vi "Set Protocol.vi"(8 "Error In":errorcluster, 10 "Protocol in":refnum<class "Protocol Parent.lvclass">, 11 "Instrument Addon Refnum In":T1 format="%.0x") -> (0 "Error Out":errorcluster, 3 "Instrument Addon Refnum Out":T1=18446744073709551615 format="%.0x")   [LabVIEW 2018, in "Instrument Addon Scripting API.lvlib"]
doc: "Sets the Protocol for the provided Instrument Addon Custom Device. \n\nThe input Protocol object must be a child of the \"Protocol\" parent class and can be an instance of the following classes: TCP.lvclass, UDP.lvclass, VISA.lvclass, RS-xxx.lvclass, AK TCP.lvclass, AK RS-xxx.lvclass, RS-xxx to GPIB ConvBox.lvclass"
uses:
  Instrument Addon Scripting API.lvlib
  <vilib>/NI Veristand/Custom Device API/Custom Device Item Ref.ctl
  Addon/Support Libraries/Protocols.lvlibp/Protocol Parent/Protocol Parent.lvclass
  Addon/Support Libraries/Protocols.lvlibp/RS-xxx/RS-xxx.lvclass
  Addon/Addon Shared/Types/RSXXX Port Settings.ctl
  Addon/Addon Shared/Types/FG Control.ctl
  Addon/Support Libraries/Protocols.lvlibp/AK RS-xxx/AK RS-xxx.lvclass
  Addon/Support Libraries/Protocols.lvlibp/UDP/UDP.lvclass
  Addon/Addon Shared/Types/UDP Settings.ctl
  Addon/Support Libraries/Protocols.lvlibp/TCP/TCP.lvclass
  Addon/Addon Shared/Types/TCPIP Settings.ctl
  Addon/Support Libraries/Protocols.lvlibp/AK TCP/AK TCP.lvclass
  Addon/Support Libraries/Protocols.lvlibp/VISA/VISA.lvclass
  Addon/Addon Shared/Types/VISA Settings.ctl
  Addon/Support Libraries/Protocols.lvlibp/RS-xxx to GPIB ConvBox/RS-xxx to GPIB ConvBox.lvclass
  Addon/Addon Shared/Types/GPIB ConvBox Settings.ctl
  Addon/Support Libraries/Protocols.lvlibp/RS-xxx/Data Access/Read PortSettings.vi
  Addon/Addon Shared/SubVIs/Constants.vi
  <vilib>/NI Veristand/Custom Device API/NI VeriStand - Get Item Property.vi
  <vilib>/NI Veristand/Custom Device API/Get Item Property (String).vi
  <vilib>/NI Veristand/Custom Device API/Get Item Property (U32).vi
  <vilib>/NI Veristand/Custom Device API/Get Item Property (Boolean).vi
  <vilib>/NI Veristand/Custom Device API/NI VeriStand - Set Item Property.vi
  <vilib>/NI Veristand/Custom Device API/Set Item Property (String).vi
  <vilib>/NI Veristand/Custom Device API/Set Item Property (U32).vi
  <vilib>/NI Veristand/Custom Device API/Set Item Property (Boolean).vi
  <vilib>/NI/NI VeriStand Advanced SysDef API/SysDef API/SysDef.Property.Get.vi
  <vilib>/NI/NI VeriStand Advanced SysDef API/_SubVIs/SysDef.Property.Get.String.vi
  <vilib>/NI/NI VeriStand Advanced SysDef API/SysDef API/SysDef.Property.Set.vi
  <vilib>/NI/NI VeriStand Advanced SysDef API/_SubVIs/SysDef.Property.Set.String.vi
  Addon/Support Libraries/Protocols.lvlibp/UDP/Data Access/Read Local IP Address.vi
  Addon/Support Libraries/Protocols.lvlibp/UDP/Data Access/Read Local Port.vi
  Addon/Support Libraries/Protocols.lvlibp/UDP/Data Access/Read Target IP Address.vi
  Addon/Support Libraries/Protocols.lvlibp/UDP/Data Access/Read Target Port.vi
  Addon/Support Libraries/Protocols.lvlibp/TCP/Data Access/Read IP Address.vi
  Addon/Support Libraries/Protocols.lvlibp/TCP/Data Access/Read Port.vi
  Addon/Support Libraries/Protocols.lvlibp/VISA/Data Access/Read Append Write Termination Character.vi
  Addon/Support Libraries/Protocols.lvlibp/VISA/Data Access/Read Enable Termination Character.vi
  Addon/Support Libraries/Protocols.lvlibp/VISA/Data Access/Read Termination Character.vi
  Addon/Support Libraries/Protocols.lvlibp/VISA/Data Access/Read Timeout.vi
  Addon/Support Libraries/Protocols.lvlibp/VISA/Data Access/Read VISA Resource.vi
  Addon/Support Libraries/Protocols.lvlibp/RS-xxx to GPIB ConvBox/Data Access/Read Assert Ren with IFC.vi
  Addon/Support Libraries/Protocols.lvlibp/RS-xxx to GPIB ConvBox/Data Access/Read ConvBox Address.vi
  Addon/Support Libraries/Protocols.lvlibp/RS-xxx to GPIB ConvBox/Data Access/Read GPIB Address.vi
  Addon/Support Libraries/Protocols.lvlibp/RS-xxx to GPIB ConvBox/Data Access/Read IST bit sense.vi
  Addon/Support Libraries/Protocols.lvlibp/RS-xxx to GPIB ConvBox/Data Access/Read Port.vi
  Addon/Support Libraries/Protocols.lvlibp/RS-xxx to GPIB ConvBox/Data Access/Read System controller.vi
  Addon/Addon Shared/Instrument Addon Shared.lvlib
  <vilib>/NI Veristand/Custom Device API/Custom Device API.lvlib
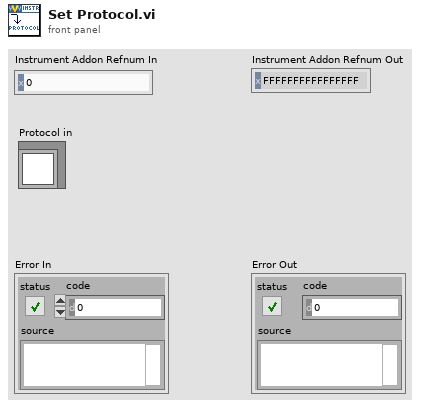
[diagram p1: front panel]
types:
  T1 = typedef "Custom Device API.lvlib/Custom Device Item Ref.ctl" = u64
  T2 = typedef "Instrument Addon Shared.lvlib/FG Control.ctl" = enum16{"Get", "Set"}
  T3 = typedef "Instrument Addon Shared.lvlib/RSXXX Port Settings.ctl" = cluster{"Port":string, "Baud Rate":u32, "Data Bits":u16, "Parity":enum16{"None", "Odd", "Even", "Mark", "Space"}, "Stop Bits":u16, "Flow Control":u16, "XON":enum16{"NUL", "SOH", "STX", "ETX", "EOT", "ENQ", "ACK", "BEL", "BS", "HT", "LF", "VT", "FF", "CR", "SO", "SI", "DLE", "DC1", "DC2", "DC3", "DC4", "NAK", "SYN", "ETB", "CAN", "EM", "SUB", "ESC", "FS", "GS", "RS", "US", "SP", "!", "\"", "#", "$", "%", "&", "'", "(", ")", "*", "+", ",", "- (-)", ".", "/", "0", "1", "2", "3", "4", "5", "6", "7", "8", "9", ":", ";", "<", "=", ">", "?", "@", "A", "B", "C", "D", "E", "F", "G", "H", "I", "J", "K", "L", "M", "N", "O", "P", "Q", "R", "S", "T", "U", "V", "W", "X", "Y", "Z", "[", "\\", "]", "^", "_", "`", "a", "b", "c", "d", "e", "f", "g", "h", "i", "j", "k", "l", "m", "n", "o", "p", "q", "r", "s", "t", "u", "v", "w", "x", "y", "z", "{", "|", "}", "~"}, "XOFF":enum16{"NUL", "SOH", "STX", "ETX", "EOT", "ENQ", "ACK", "BEL", "BS", "HT", "LF", "VT", "FF", "CR", "SO", "SI", "DLE", "DC1", "DC2", "DC3", "DC4", "NAK", "SYN", "ETB", "CAN", "EM", "SUB", "ESC", "FS", "GS", "RS", "US", "SP", "!", "\"", "#", "$", "%", "&", "'", "(", ")", "*", "+", ",", "- (-)", ".", "/", "0", "1", "2", "3", "4", "5", "6", "7", "8", "9", ":", ";", "<", "=", ">", "?", "@", "A", "B", "C", "D", "E", "F", "G", "H", "I", "J", "K", "L", "M", "N", "O", "P", "Q", "R", "S", "T", "U", "V", "W", "X", "Y", "Z", "[", "\\", "]", "^", "_", "`", "a", "b", "c", "d", "e", "f", "g", "h", "i", "j", "k", "l", "m", "n", "o", "p", "q", "r", "s", "t", "u", "v", "w", "x", "y", "z", "{", "|", "}", "~"}, "End Read on Termination Character":bool, "End Write on Termination Character":bool, "Termination Character":u8}
  T4 = typedef "Instrument Addon Shared.lvlib/UDP Settings.ctl" = cluster{"Local IP Address":string, "Local Port":u16, "Target IP Address":string, "Target Port":u16}
  T5 = typedef "Instrument Addon Shared.lvlib/TCPIP Settings.ctl" = cluster{"IP Address":string, "Port":u16}
  T6 = typedef "Instrument Addon Shared.lvlib/VISA Settings.ctl" = cluster{"VISA Resource":string, "Enable Termination Character":bool, "Termination Character":u8, "Timeout":u32, "Append Write Termination Character":bool}
  T7 = typedef "Instrument Addon Shared.lvlib/GPIB ConvBox Settings.ctl" = cluster{"Port":string, "ConvBox Address":string, "Assert Ren with IFC":bool, "System controller":bool, "IST bit sense":bool, "GPIB Address":string}
  T8 = typedef "Protocols.lvlibp/Protocol Parent.lvclass/Base Protocol Type.ctl" = enum16{"RS-XXX", "VISA", "TCPIP", "UDP", "GPIB ConvBox"}
  T9 = cluster{"Port":string, "Baud Rate":u32, "Data Bits":u16, "Parity":enum16{"None", "Odd", "Even", "Mark", "Space"}, "Stop Bits":u16, "Flow Control":u16, "XON":enum16{"NUL", "SOH", "STX", "ETX", "EOT", "ENQ", "ACK", "BEL", "BS", "HT", "LF", "VT", "FF", "CR", "SO", "SI", "DLE", "DC1", "DC2", "DC3", "DC4", "NAK", "SYN", "ETB", "CAN", "EM", "SUB", "ESC", "FS", "GS", "RS", "US", "SP", "!", "\"", "#", "$", "%", "&", "'", "(", ")", "*", "+", ",", "- (-)", ".", "/", "0", "1", "2", "3", "4", "5", "6", "7", "8", "9", ":", ";", "<", "=", ">", "?", "@", "A", "B", "C", "D", "E", "F", "G", "H", "I", "J", "K", "L", "M", "N", "O", "P", "Q", "R", "S", "T", "U", "V", "W", "X", "Y", "Z", "[", "\\", "]", "^", "_", "`", "a", "b", "c", "d", "e", "f", "g", "h", "i", "j", "k", "l", "m", "n", "o", "p", "q", "r", "s", "t", "u", "v", "w", "x", "y", "z", "{", "|", "}", "~"}, "XOFF":enum16{"NUL", "SOH", "STX", "ETX", "EOT", "ENQ", "ACK", "BEL", "BS", "HT", "LF", "VT", "FF", "CR", "SO", "SI", "DLE", "DC1", "DC2", "DC3", "DC4", "NAK", "SYN", "ETB", "CAN", "EM", "SUB", "ESC", "FS", "GS", "RS", "US", "SP", "!", "\"", "#", "$", "%", "&", "'", "(", ")", "*", "+", ",", "- (-)", ".", "/", "0", "1", "2", "3", "4", "5", "6", "7", "8", "9", ":", ";", "<", "=", ">", "?", "@", "A", "B", "C", "D", "E", "F", "G", "H", "I", "J", "K", "L", "M", "N", "O", "P", "Q", "R", "S", "T", "U", "V", "W", "X", "Y", "Z", "[", "\\", "]", "^", "_", "`", "a", "b", "c", "d", "e", "f", "g", "h", "i", "j", "k", "l", "m", "n", "o", "p", "q", "r", "s", "t", "u", "v", "w", "x", "y", "z", "{", "|", "}", "~"}, "End Read on Termination Character":bool, "End Write on Termination Character":bool, "Termination Character":u8}
  T10 = enum16{"NUL", "SOH", "STX", "ETX", "EOT", "ENQ", "ACK", "BEL", "BS", "HT", "LF", "VT", "FF", "CR", "SO", "SI", "DLE", "DC1", "DC2", "DC3", "DC4", "NAK", "SYN", "ETB", "CAN", "EM", "SUB", "ESC", "FS", "GS", "RS", "US", "SP", "!", "\"", "#", "$", "%", "&", "'", "(", ")", "*", "+", ",", "- (-)", ".", "/", "0", "1", "2", "3", "4", "5", "6", "7", "8", "9", ":", ";", "<", "=", ">", "?", "@", "A", "B", "C", "D", "E", "F", "G", "H", "I", "J", "K", "L", "M", "N", "O", "P", "Q", "R", "S", "T", "U", "V", "W", "X", "Y", "Z", "[", "\\", "]", "^", "_", "`", "a", "b", "c", "d", "e", "f", "g", "h", "i", "j", "k", "l", "m", "n", "o", "p", "q", "r", "s", "t", "u", "v", "w", "x", "y", "z", "{", "|", "}", "~"}
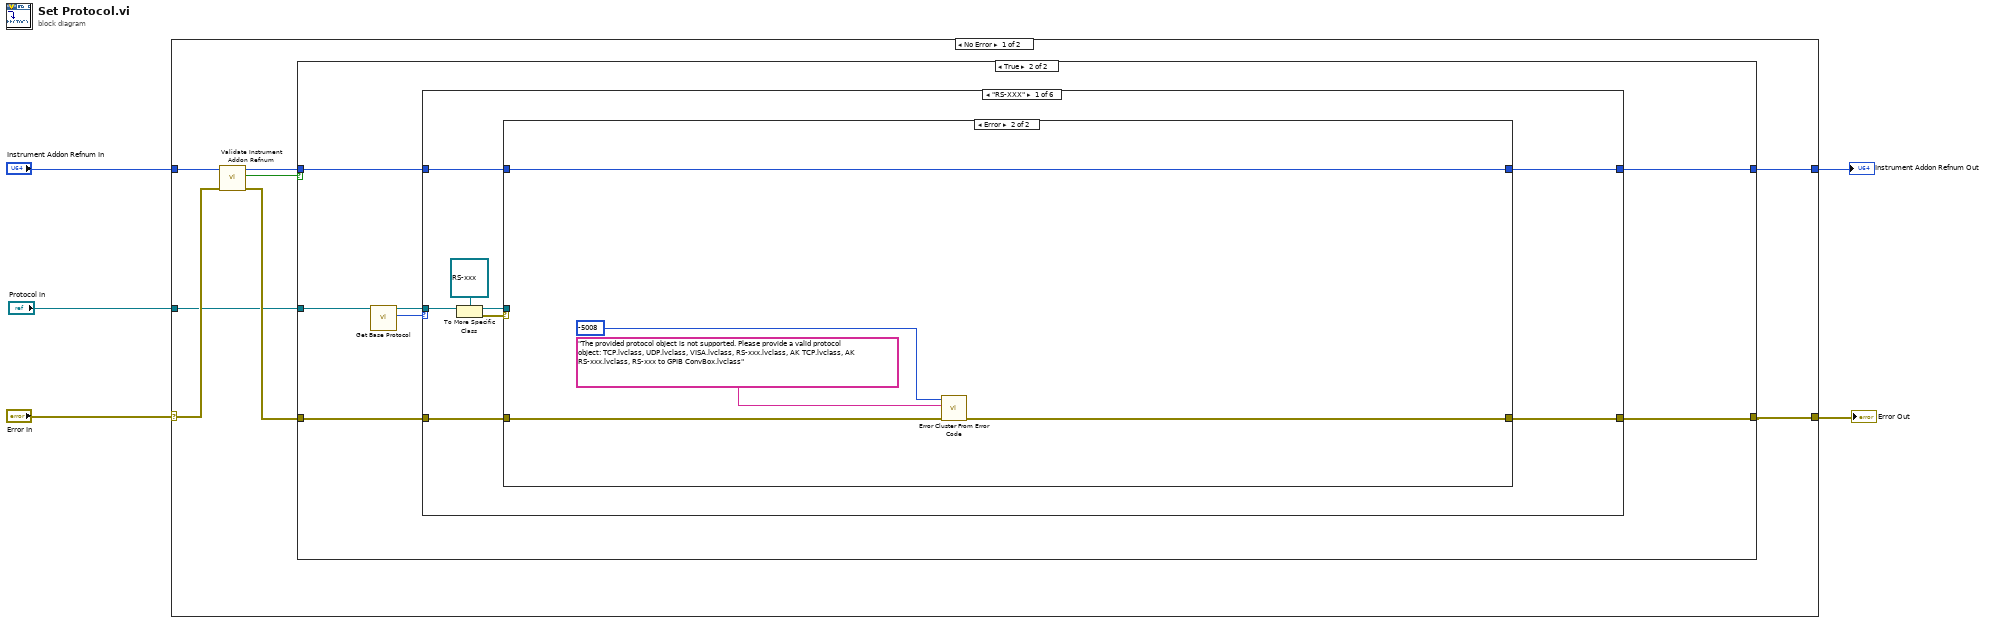
[diagram p0: block diagram]
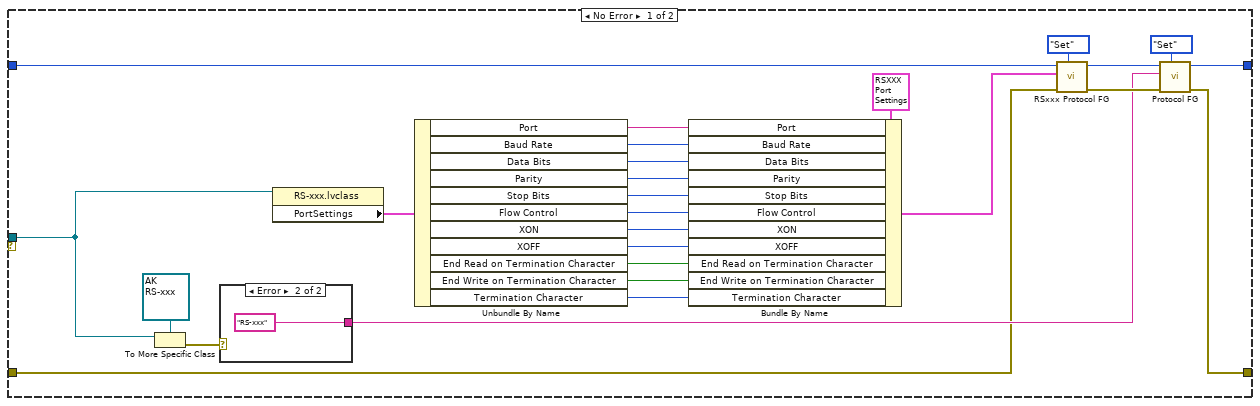
[diagram p3: hidden frame]
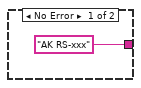
[diagram p4: hidden frame]
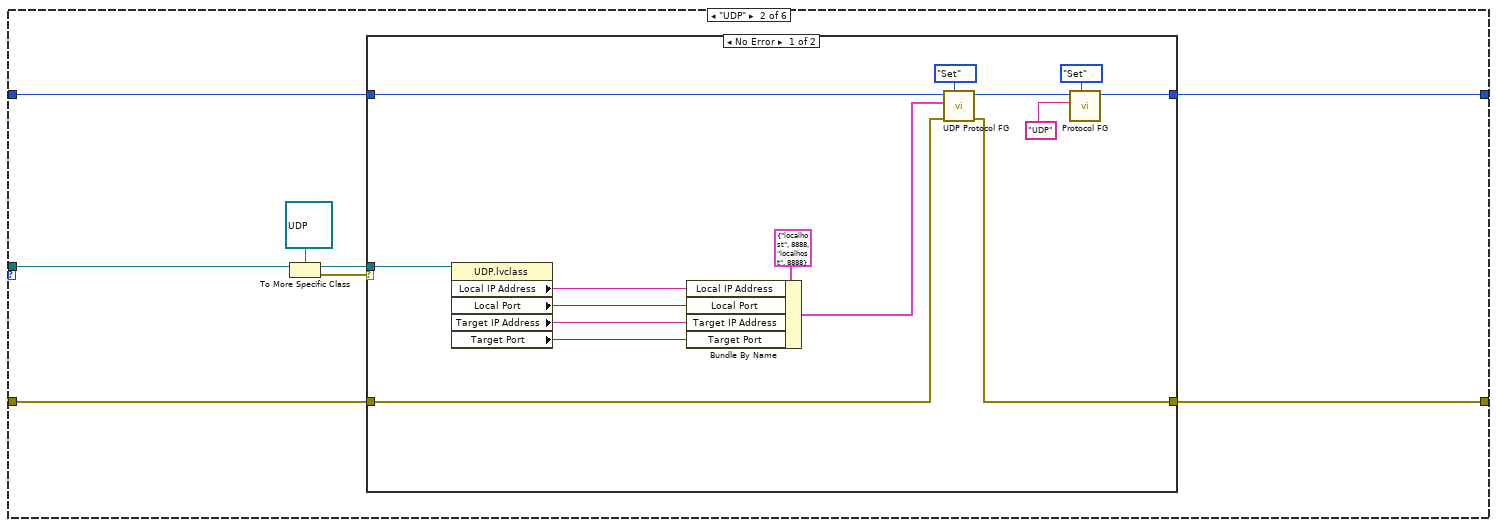
[diagram p5: hidden frame]
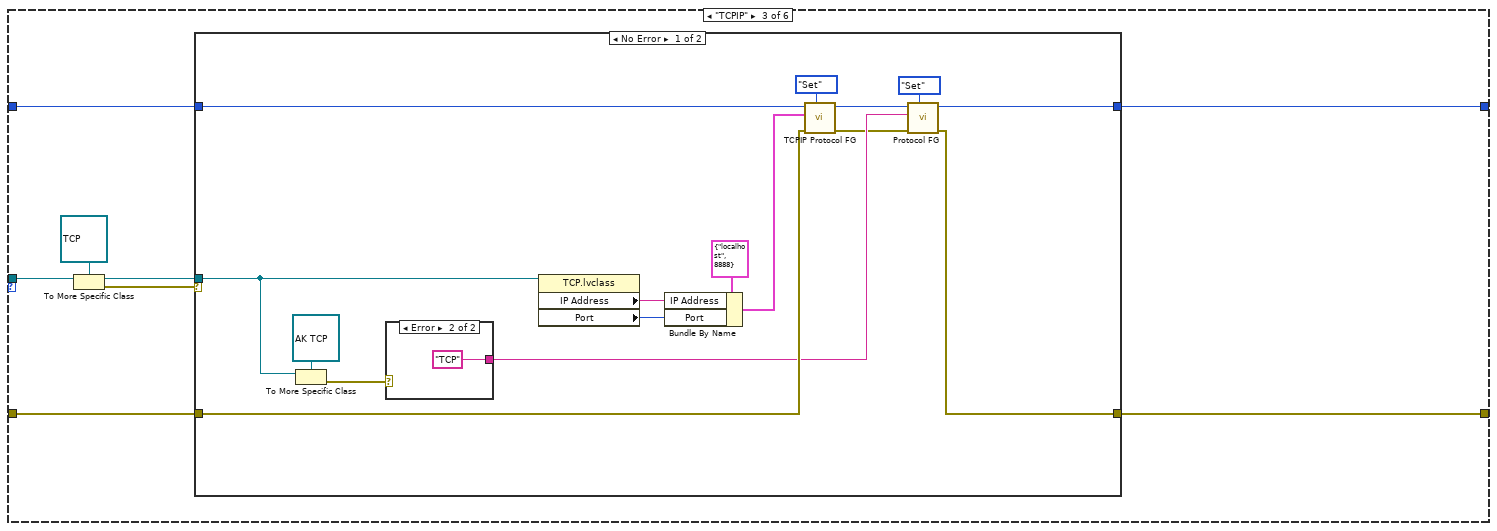
[diagram p7: hidden frame]
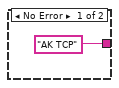
[diagram p8: hidden frame]
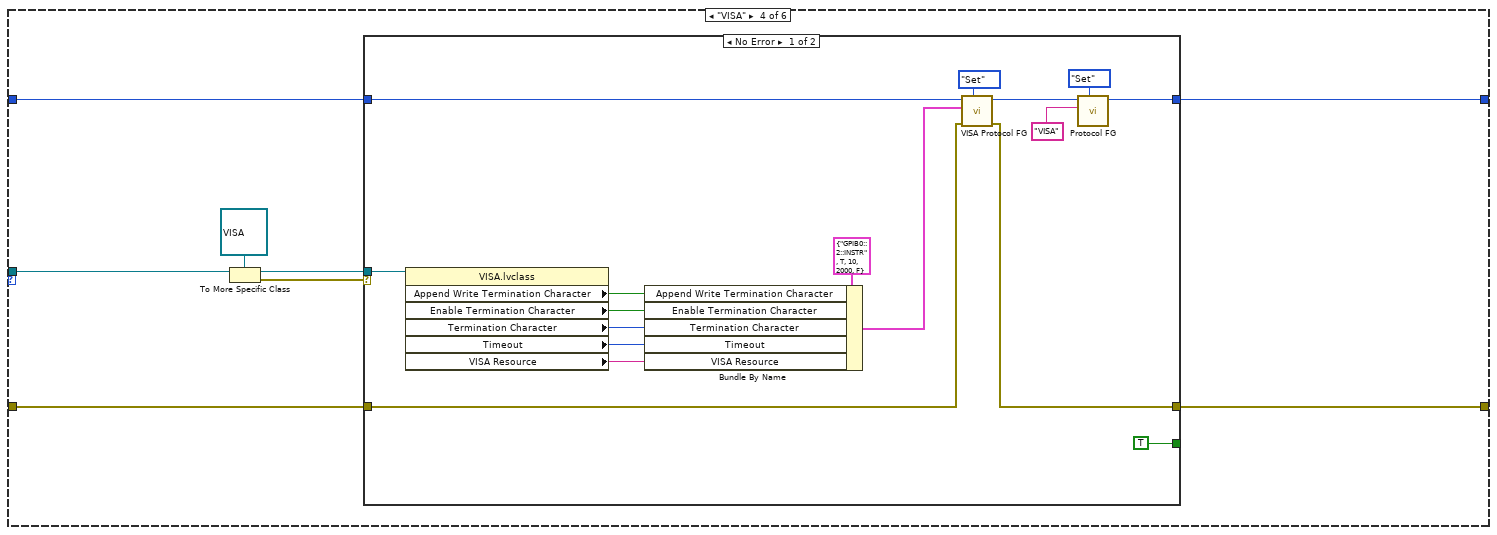
[diagram p10: hidden frame]
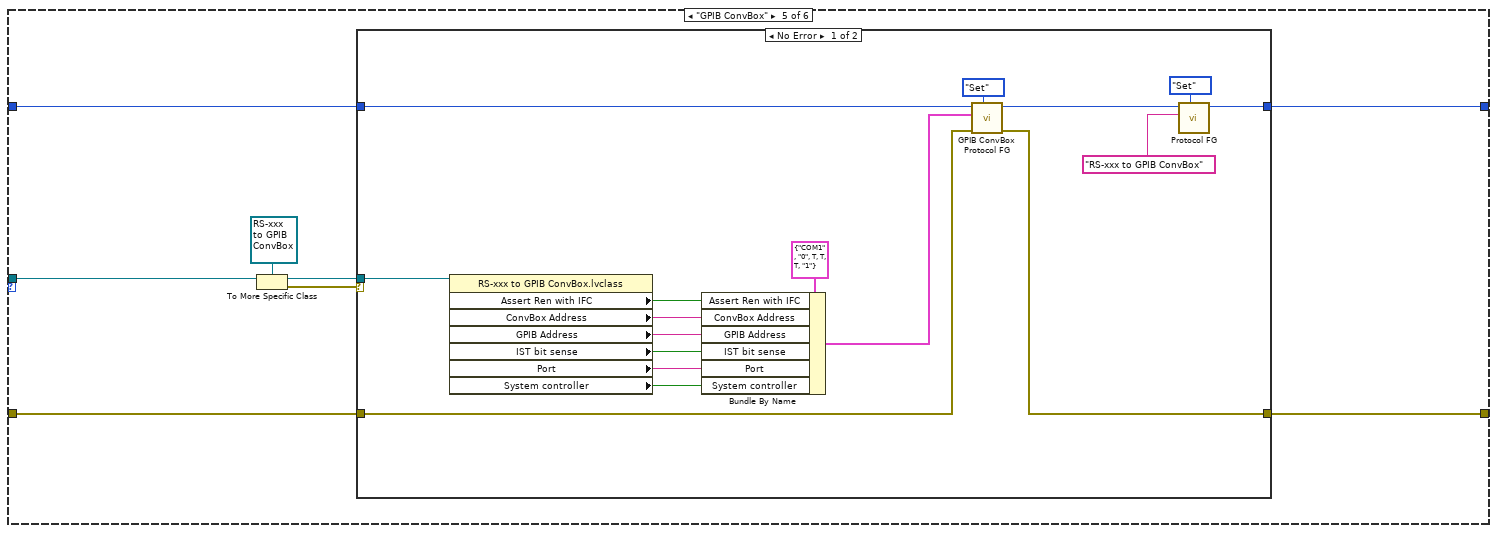
[diagram p12: hidden frame]
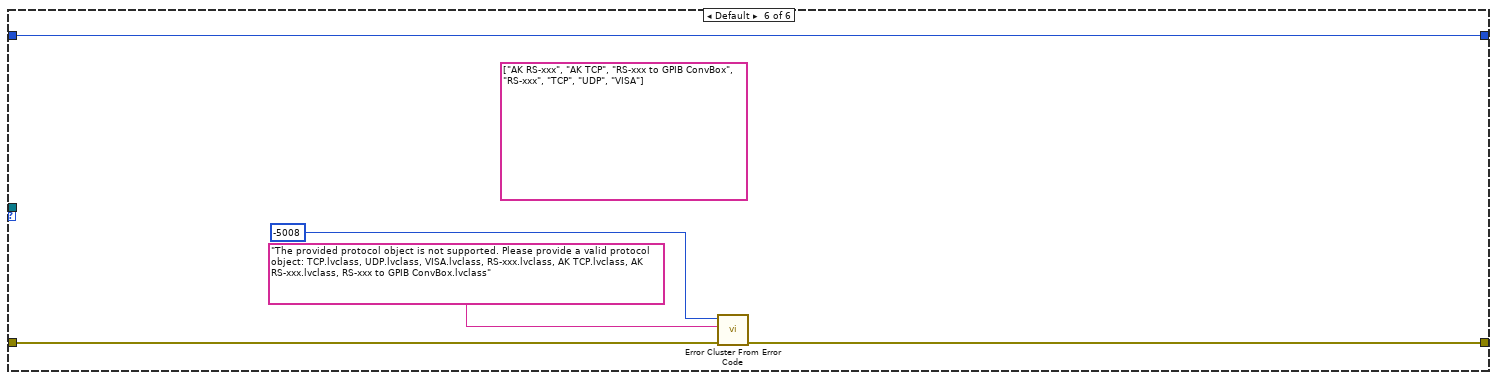
[diagram p14: hidden frame]
diagram:
  n1 = case shown="No Error" "Error In" {
    selector: "Error In" -> [w12 w177]
    tunnel: "Instrument Addon Refnum In" -> [w13 w176]
    tunnel: [w9 w177] -> w4
    tunnel: [w8 w176] -> w2
    tunnel: "Protocol in" -> [w6 _]
    frame No Error {
      n2 = call "Validate Instrument Addon Refnum.vi"("Error In"=w12, "Refnum In"=w13) -> ("Error Out"=w7:errorcluster, "Is Instrument Addon?"=w10:bool, "Refnum Out"=w11:T1)  [unwired: 7 in]
      n3 = case shown="True" w10 {
        tunnel: w11 -> [w15 w21]
        tunnel: [w14 w19] -> w9
        tunnel: [w15 w20] -> w8
        tunnel: w7 -> [w14 w22]
        tunnel: w6 -> [_ w18]
        frame False {
        }
        frame True {
          n4 = call-dynamic "Get Base Protocol.vi"("Protocol Parent in"=w18) -> ("Protocol out"=w16:T8, "Protocol Parent out"=w17:refnum<class "Protocol Parent.lvclass">)  [unwired: 8 in, 1 out]
          n5 = case shown="\"RS-XXX\"" w16 {
            tunnel: w17 -> [w29 w71 w96 w124 w151 _]
            tunnel: w22 -> [w24 w65 w90 w121 w147 w174]
            tunnel: w21 -> [w26 w69 w92 w120 w146 w175]
            tunnel: [w25 w68 w91 w118 w145 w175] -> w20
            tunnel: [w23 w64 w89 w117 w144 w171] -> w19
            frame "RS-XXX" {
              n6 = To More Specific Class(target class=refnum<class "RS-xxx.lvclass"> refnum ("Protocols.lvlibp:RS-xxx.lvclass"), reference=w29) -> (specific class reference=w27:refnum<class "RS-xxx.lvclass">, error out=w28:errorcluster)  [unwired: 1 in]
              n7 = case shown="Error" w28 {
                tunnel: w27 -> [w34 _]
                tunnel: w26 -> [w54 w63]
                tunnel: [w37 w63] -> w25
                tunnel: w24 -> [w31 w60]
                tunnel: [w36 w59] -> w23
                frame No Error {
                  n8 = To More Specific Class(target class=refnum<class "AK RS-xxx.lvclass"> refnum ("Protocols.lvlibp:AK RS-xxx.lvclass"), reference=w34) -> (error out=w33:errorcluster)  [unwired: 1 in, 1 out]
                  n9 = case shown="Error" w33 {
                    tunnel: ["AK RS-xxx" ("filename without extension") "RS-xxx" ("filename without extension")] -> w32
                    frame No Error {
                    }
                    frame Error {
                    }
                  }
                  n10 = property class="RS-xxx.lvclass"(reference=w34) -> ("PortSettings"=w55:T9)  [unwired: 1 in, 2 out]
                  n11 = Unbundle By Name(w55) -> ("Port"=w53:string, "Baud Rate"=w52:u32, "Data Bits"=w51:u16, "Parity"=w50:enum16{"None", "Odd", "Even", "Mark", "Space"}, "Stop Bits"=w49:u16, "Flow Control"=w48:u16, "XON"=w47:T10, "XOFF"=w46:T10, "End Read on Termination Character"=w45:bool, "End Write on Termination Character"=w44:bool, "Termination Character"=w43:u8)
                  n12 = Bundle By Name(cluster=T3 {"Port"="COM1", "Baud Rate"=9600, "Data Bits"=8, "Parity"=enum."None", "Stop Bits"=10, "Flow Control"=0, "XON"=enum."DC1", "XOFF"=enum."DC3", "End Read on Termination Character"=TRUE, "End Write on Termination Character"=TRUE, "Termination Character"=10} ("Serial Config"), "Port"=w53, "Baud Rate"=w52, "Data Bits"=w51, "Parity"=w50, "Stop Bits"=w49, "Flow Control"=w48, "XON"=w47, "XOFF"=w46, "End Read on Termination Character"=w45, "End Write on Termination Character"=w44, "Termination Character"=w43) -> (w41:T3)
                  n13 = call "RSxxx Protocol FG.vi"("Action"=FG_Control."Set", "error in (no error)"=w31, "Serial Config"=w41, "Device Item Ref in"=w54) -> ("error out"=w38:errorcluster, "Item Ref out"=w39:T1)  [unwired: 5 in, 1 out]
                  n14 = call "Protocol FG.vi"("Action"=FG_Control."Set", "error in (no error)"=w38, "Protocol"=w32, "Device Item Ref in"=w39) -> ("error out"=w36:errorcluster, "Item Ref out"=w37:T1)  [unwired: 5 in, 1 out]
                }
                frame Error {
                  n15 = call <vilib>:"Error Cluster From Error Code.vi"("error in (no error)"=w60, "error message (\"\")"="The provided protocol object is not supported. Please provide a valid protocol object: TCP.lvclass, UDP.lvclass, VISA.lvclass, RS-xxx.lvclass, AK TCP.lvclass, AK RS-xxx.lvclass, RS-xxx to GPIB ConvBox.lvclass" ("error message (\"\")"), "error code (0)"=-5008) -> ("error out"=w59:errorcluster)  [unwired: 6 in]
                }
              }
            }
            frame "UDP" {
              n16 = To More Specific Class(target class=refnum<class "UDP.lvclass"> refnum ("Protocols.lvlibp:UDP.lvclass"), reference=w71) -> (specific class reference=w66:refnum<class "UDP.lvclass">, error out=w67:errorcluster)  [unwired: 1 in]
              n17 = case shown="No Error" w67 {
                tunnel: w69 -> [w86 w88]
                tunnel: [w73 w88] -> w68
                tunnel: w66 -> [w84 _]
                tunnel: w65 -> [w77 w87]
                tunnel: [w76 w87] -> w64
                frame No Error {
                  n18 = property class="UDP.lvclass"(reference=w84) -> ("Local IP Address"=w82:string, "Local Port"=w81:u16, "Target IP Address"=w80:string, "Target Port"=w79:u16)  [unwired: 1 in, 2 out]
                  n19 = Bundle By Name(cluster=T4 {"Local IP Address"="localhost", "Local Port"=8888, "Target IP Address"="localhost", "Target Port"=8888} ("UDP Config"), "Local IP Address"=w82, "Local Port"=w81, "Target IP Address"=w80, "Target Port"=w79) -> (w78:T4)
                  n20 = call "UDP Protocol FG.vi"("Action"=FG_Control."Set", "error in (no error)"=w77, "UDP Config"=w78, "Device Item Ref in"=w86) -> ("error out"=w76:errorcluster, "Item Ref out"=w74:T1)  [unwired: 5 in, 1 out]
                  n21 = call "Protocol FG.vi"("Action"=FG_Control."Set", "Protocol"="UDP" ("Local IP Address"), "Device Item Ref in"=w74) -> ("Item Ref out"=w73:T1)  [unwired: 6 in, 2 out]
                }
                frame Error {
                }
              }
            }
            frame "TCPIP" {
              n22 = To More Specific Class(target class=refnum<class "TCP.lvclass"> refnum ("Protocols.lvlibp:TCP.lvclass"), reference=w96) -> (specific class reference=w93:refnum<class "TCP.lvclass">, error out=w94:errorcluster)  [unwired: 1 in]
              n23 = case shown="No Error" w94 {
                tunnel: w93 -> [w103 _]
                tunnel: w92 -> [w107 w115]
                tunnel: [w100 w115] -> w91
                tunnel: w90 -> [w106 w116]
                tunnel: [w97 w116] -> w89
                frame No Error {
                  n24 = To More Specific Class(target class=refnum<class "AK TCP.lvclass"> refnum ("Protocols.lvlibp:AK TCP.lvclass"), reference=w103) -> (error out=w105:errorcluster)  [unwired: 1 in, 1 out]
                  n25 = case shown="Error" w105 {
                    tunnel: ["AK TCP" ("filename without extension") "TCP" ("filename without extension")] -> w99
                    frame No Error {
                    }
                    frame Error {
                    }
                  }
                  n26 = property class="TCP.lvclass"(reference=w103) -> ("IP Address"=w110:string, "Port"=w109:u16)  [unwired: 1 in, 2 out]
                  n27 = Bundle By Name(cluster=T5 {"IP Address"="localhost", "Port"=8888} ("TCP/IP Config"), "IP Address"=w110, "Port"=w109) -> (w108:T5)
                  n28 = call "TCPIP Protocol FG.vi"("Action"=FG_Control."Set", "error in (no error)"=w106, "TCP/IP Config"=w108, "Device Item Ref in"=w107) -> ("error out"=w98:errorcluster, "Item Ref out"=w101:T1)  [unwired: 5 in, 1 out]
                  n29 = call "Protocol FG.vi"("Action"=FG_Control."Set", "error in (no error)"=w98, "Protocol"=w99, "Device Item Ref in"=w101) -> ("error out"=w97:errorcluster, "Item Ref out"=w100:T1)  [unwired: 5 in, 1 out]
                }
                frame Error {
                }
              }
            }
            frame "VISA" {
              n30 = To More Specific Class(target class=refnum<class "VISA.lvclass"> refnum ("Protocols.lvlibp:VISA.lvclass"), reference=w124) -> (specific class reference=w119:refnum<class "VISA.lvclass">, error out=w122:errorcluster)  [unwired: 1 in]
              n31 = case shown="No Error" w122 {
                tunnel: w121 -> [w130 w142]
                tunnel: w120 -> [w140 w143]
                tunnel: w119 -> [w141 _]
                tunnel: [w126 w143] -> w118
                tunnel: [TRUE _] -> _
                tunnel: [w129 w142] -> w117
                frame No Error {
                  n32 = property class="VISA.lvclass"(reference=w141) -> ("Append Write Termination Character"=w137:bool, "Enable Termination Character"=w136:bool, "Termination Character"=w135:u8, "Timeout"=w134:u32, "VISA Resource"=w133:string)  [unwired: 1 in, 2 out]
                  n33 = Bundle By Name(cluster=T6 {"VISA Resource"="GPIB0::2::INSTR", "Enable Termination Character"=TRUE, "Termination Character"=10, "Timeout"=2000, "Append Write Termination Character"=FALSE} ("VISA Config"), "Append Write Termination Character"=w137, "Enable Termination Character"=w136, "Termination Character"=w135, "Timeout"=w134, "VISA Resource"=w133) -> (w132:T6)
                  n34 = call "VISA Protocol FG.vi"("Action"=FG_Control."Set", "error in (no error)"=w130, "VISA Config"=w132, "Device Item Ref in"=w140) -> ("error out"=w129:errorcluster, "Item Ref out"=w127:T1)  [unwired: 5 in, 1 out]
                  n35 = call "Protocol FG.vi"("Action"=FG_Control."Set", "Protocol"="VISA", "Device Item Ref in"=w127) -> ("Item Ref out"=w126:T1)  [unwired: 6 in, 2 out]
                }
                frame Error {
                }
              }
            }
            frame "GPIB ConvBox" {
              n36 = To More Specific Class(target class=refnum<class "RS-xxx to GPIB ConvBox.lvclass"> refnum ("Protocols.lvlibp:RS-xxx to GPIB ConvBox.lvclass"), reference=w151) -> (specific class reference=w148:refnum<class "RS-xxx to GPIB ConvBox.lvclass">, error out=w149:errorcluster)  [unwired: 1 in]
              n37 = case shown="No Error" w149 {
                tunnel: w148 -> [w168 _]
                tunnel: w147 -> [w166 w170]
                tunnel: w146 -> [w157 w169]
                tunnel: [w152 w169] -> w145
                tunnel: [w156 w170] -> w144
                frame No Error {
                  n38 = property class="RS-xxx to GPIB ConvBox.lvclass"(reference=w168) -> ("Assert Ren with IFC"=w164:bool, "ConvBox Address"=w163:string, "GPIB Address"=w162:string, "IST bit sense"=w161:bool, "Port"=w160:string, "System controller"=w159:bool)  [unwired: 1 in, 2 out]
                  n39 = Bundle By Name(cluster=T7 {"Port"="COM1", "ConvBox Address"="0", "Assert Ren with IFC"=TRUE, "System controller"=TRUE, "IST bit sense"=TRUE, "GPIB Address"="1"} ("GPIB ConvBox Config"), "Assert Ren with IFC"=w164, "ConvBox Address"=w163, "GPIB Address"=w162, "IST bit sense"=w161, "Port"=w160, "System controller"=w159) -> (w158:T7)
                  n40 = call "GPIB ConvBox Protocol FG.vi"("Action"=FG_Control."Set", "error in (no error)"=w166, "GPIB ConvBox Config"=w158, "Device Item Ref in"=w157) -> ("error out"=w156:errorcluster, "Item Ref out"=w153:T1)  [unwired: 5 in, 1 out]
                  n41 = call "Protocol FG.vi"("Action"=FG_Control."Set", "Protocol"="RS-xxx to GPIB ConvBox", "Device Item Ref in"=w153) -> ("Item Ref out"=w152:T1)  [unwired: 6 in, 2 out]
                }
                frame Error {
                }
              }
            }
            frame Default {
              (unwired) string[] ["AK RS-xxx", "AK TCP", "RS-xxx to GPIB ConvBox", "RS-xxx", "TCP", "UDP", "VISA"] ("Array")
              n42 = call <vilib>:"Error Cluster From Error Code.vi"("error in (no error)"=w174, "error message (\"\")"="The provided protocol object is not supported. Please provide a valid protocol object: TCP.lvclass, UDP.lvclass, VISA.lvclass, RS-xxx.lvclass, AK TCP.lvclass, AK RS-xxx.lvclass, RS-xxx to GPIB ConvBox.lvclass" ("error message (\"\")"), "error code (0)"=-5008) -> ("error out"=w171:errorcluster)  [unwired: 6 in]
            }
          }
        }
      }
    }
    frame Error {
    }
  }
  "Error Out" <- w4
  "Instrument Addon Refnum Out" <- w2
